vi "AutoDriveStraight.vi"(8 "error in (no error)":errorcluster, 9 "TimeOut (s)":dbl=99.0, 10 "MaxSpeed (ft/s)":dbl, 11 "Dist (ft)":dbl) -> (0 "error out":errorcluster)   [LabVIEW 2023]
doc: "Wrapper class for drive straight"
uses:
  <vilib>/Rock Robotics/WPI/ThirdParty/JAS_Junk/TrajLib/ChassisSpeeds_New.vi
  <vilib>/Rock Robotics/WPI/ThirdParty/JAS_Junk/TrajLib/Conv_Feet_Meters.vi
  <vilib>/Rock Robotics/WPI/ThirdParty/JAS_Junk/TrajLib/Conv_Deg_Radians.vi
  <vilib>/Utility/semaphor.llb/Obtain Semaphore Reference.vi
  <vilib>/Rock Robotics/WPI/ThirdParty/JAS_Junk/TrajLib/Timer_Reset.vi
  Drive/DriveGlobal.vi
  <vilib>/Rock Robotics/WPI/ThirdParty/JAS_Junk/TrajLib/Trajectory_Library.lvlib
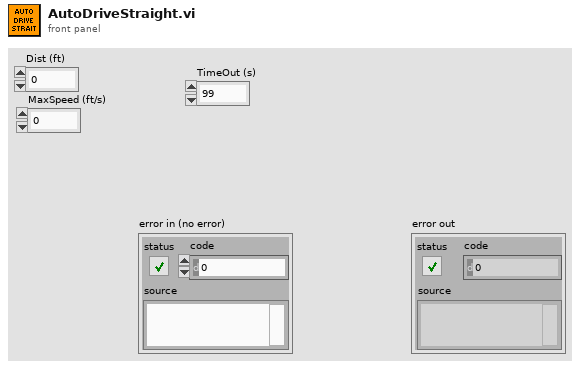
[diagram p1: front panel]
types:
  T1 = typedef "Trajectory_Library.lvlib/TIMER.ctl" = cluster{"StartTime":dbl, "Accumulated TIme":dbl, "Running":bool, "semaphore":T2}
  T2 = typedef "Semaphore RefNum" = refnum<k1>
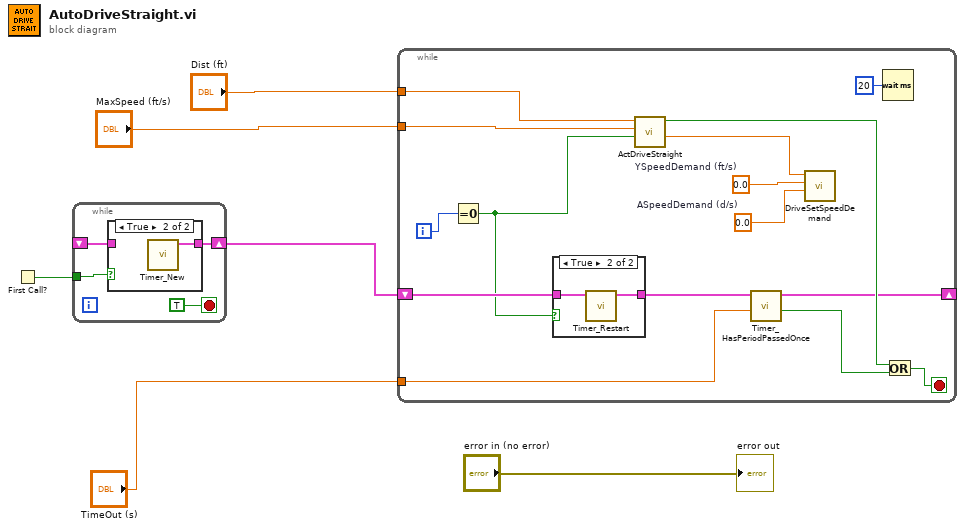
[diagram p0: block diagram]
diagram:
  n1 = First Call?() -> (First Call?: T/F=w2:bool)
  n2 = while {
    tunnel: w2 -> [w7]
    shift-right: [w10] -> w1
    shift-left: _ -> [w8]
    stop <- TRUE stop-if-true
    n3 = case shown="True" w7 {
      tunnel: [w11 w12] -> w10
      tunnel: w8 -> [w11 _]
      frame False {
      }
      frame True {
        n4 = call <vilib>:"Timer_New.vi"() -> ("TIMER"=w12:T1)  [unwired: 11 in]
      }
    }
  }
  n5 = while {
    tunnel: "Dist (ft)" -> [w27]
    tunnel: "MaxSpeed (ft/s)" -> [w26]
    tunnel: "TimeOut (s)" -> [w24]
    shift-right: [w14] -> _
    shift-left: w1 -> [w16]
    i -> [w25]
    stop <- w22 stop-if-true
    w17 = 0.0  # ASpeedDemand (d/s)
    w18 = 0.0  # YSpeedDemand (ft/s)
    n6 = Equal To 0?(x=w25) -> (x = 0?=w13:bool)
    n7 = case shown="True" w13 {
      tunnel: w16 -> [w28 w30]
      tunnel: [w28 w29] -> w15
      frame False {
      }
      frame True {
        n8 = call <vilib>:"Timer_Restart.vi"("in Timer"=w30) -> ("out Timer"=w29:T1)  [unwired: 10 in]
      }
    }
    n9 = call "ActDriveStraight.vi"("FirstTime"=w13, "MaxSpeed (ft/s)"=w26, "Dist (ft)"=w27) -> ("XSpeedDemand"=w19:dbl, "Done"=w21:bool)  [unwired: 7 in]
    n10 = call <vilib>:"Timer_HasPeriodPassedOnce.vi"("Period"=w24, "in Timer"=w15) -> ("Expired"=w23:bool, "out Timer"=w14:T1)  [unwired: 7 in, 1 out]
    n11 = call "DriveSetSpeedDemand.vi"("ASpeedDemand (d/s)"=w17, "YSpeedDemand (ft/s)"=w18, "XSpeedDemand (ft/s)"=w19) -> ()  [unwired: 9 in]
    n12 = Wait (ms)(milliseconds to wait=u32 20) -> ()  [unwired: 1 out]
    n13 = Or(x=w21, y=w23) -> (x .or. y?=w22:bool)
  }
  "error out" <- "error in (no error)"
